vi "VG-requestCalibration.vi"(8 "error in (no error)":errorcluster, 10 "Calibration Type":T1=enum."Short", 11 "VG-VNA_GUI in":refnum<class "VG-VNA_GUI.lvclass">) -> (0 "error out":errorcluster, 3 "VG-VNA_GUI out":refnum<class "VG-VNA_GUI.lvclass">)   [LabVIEW 2020, in "VG-VNA_GUI.lvlib" / "VG-VNA_GUI.lvclass"]
uses:
  VG-VNA_GUI.lvclass
  data_handler/VDH-VNA_data_handler/VDH-VNA_data_handler/VDH-Calibration_enum.ctl
  VG-VNA_GUI.lvclass/VG-VNA_GUI.ctl
  data_handler/VDH-VNA_data_handler/VDH-VNA_data_handler Messages/VDH-RequestCalibration Msg/VDH-RequestCalibration Msg.lvclass/VDH-RequestCalibration Msg.ctl
  <vilib>/ActorFramework/Message Enqueuer/Message Enqueuer.lvclass/Message Enqueuer.ctl
  <vilib>/ActorFramework/Message Enqueuer/Enqueue.vi
  data_handler/VDH-VNA_data_handler/VDH-VNA_data_handler Messages/VDH-RequestCalibration Msg/VDH-RequestCalibration Msg.lvclass
  C:/Program Files (x86)/National Instruments/LabVIEW 2020/vi.lib/ActorFramework/Message/Message.lvclass
  <vilib>/ActorFramework/Message Priority Queue/Priority Enqueue.vi
  data_handler/VDH-VNA_data_handler/VDH-VNA_data_handler/VDH-VNA_data_handler.lvclass
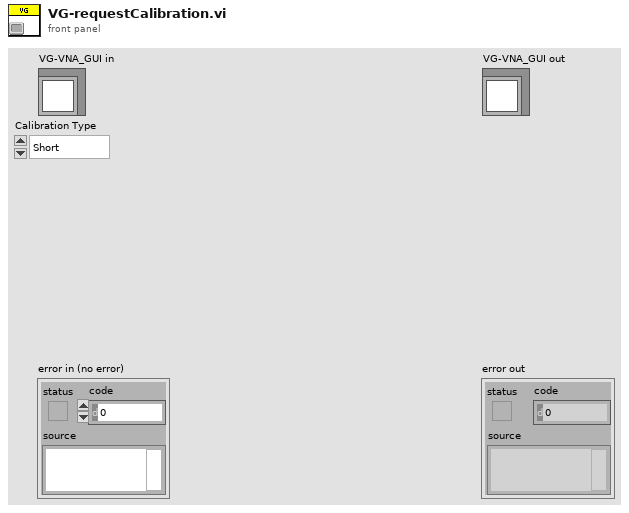
[diagram p1: front panel]
types:
  T1 = typedef "VDH-VNA_data_handler.lvlib/VDH-VNA_data_handler.lvclass/VDH-Calibration_enum.ctl" = enum16{"Non", "Short", "Open", "Load", "Through", "Permativity"}
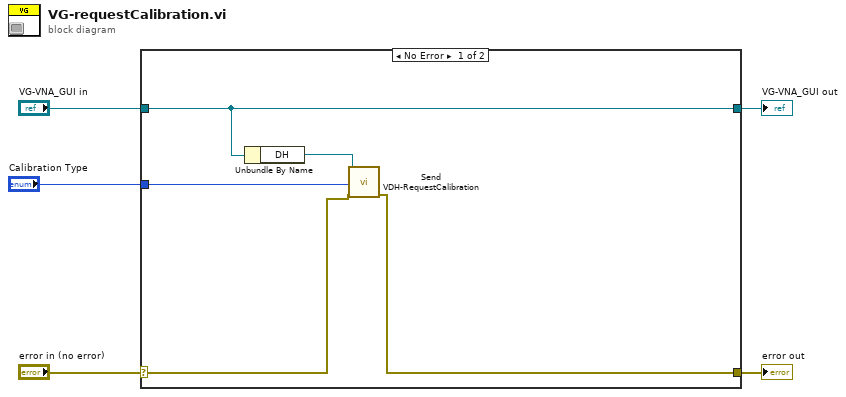
[diagram p0: block diagram]
diagram:
  n1 = case shown="No Error" "error in (no error)" {
    selector: "error in (no error)" -> [w7 w12]
    tunnel: [w6 w12] -> w4
    tunnel: [w10 w11] -> w2
    tunnel: "VG-VNA_GUI in" -> [w10 w11]
    tunnel: "Calibration Type" -> [w8 _]
    frame No Error {
      n2 = Unbundle By Name(w10) -> ("DH"=w9:refnum<class "Message Enqueuer.lvclass">)
      n3 = call "Send VDH-RequestCalibration.vi"("error in (no error)"=w7, "Calibration Type"=w8, "Message Enqueuer"=w9) -> ("error out"=w6:errorcluster)  [unwired: 7 in, 1 out]
    }
    frame Error {
    }
  }
  "error out" <- w4
  "VG-VNA_GUI out" <- w2
